vi "Is_Atomic_Parent.vi"(8 "error in (no error)":errorcluster, 11 "AB_Source_Container in":refnum<class "AB_Source_Container.lvclass">) -> (0 "error out":errorcluster, 1 "autoAdd":bool, 2 "atomicContainer":bool, 3 "AB_Source_Container out":refnum<class "AB_Source_Container.lvclass">)   [LabVIEW 2020, in "AB_Source_Container.lvclass"]
uses:
  <vilib>/AppBuilder/AB_Classes/Source/Container/AB_Source_Container.lvclass
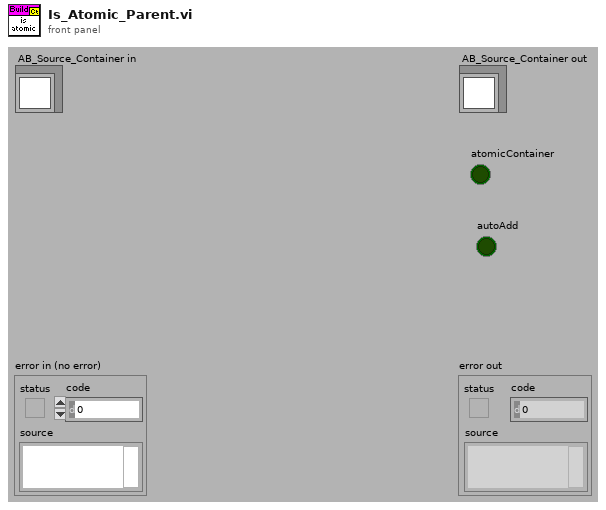
[diagram p1: front panel]
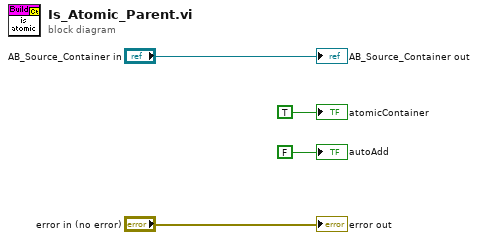
[diagram p0: block diagram]
diagram:
  "error out" <- "error in (no error)"
  "atomicContainer" <- TRUE ("atomicContainer")
  "AB_Source_Container out" <- "AB_Source_Container in"
  "autoAdd" <- FALSE ("autoAdd")
